vi "Buttons enable or disable.vi"(8 "error in (no error)":errorcluster, 10 "Enabled or Disabled?":T1(ring), 11 "Input references array":refnum<vi>[](array[refnum])) -> (0 "error out":errorcluster)   [LabVIEW 2014]
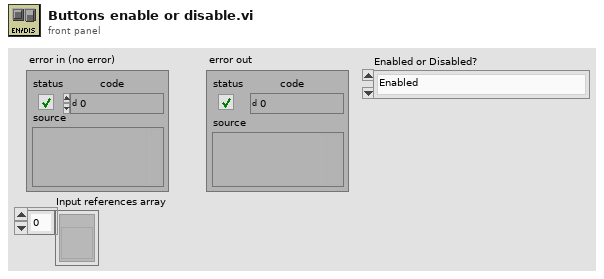
[diagram p1: front panel]
types:
  T1 = enum8{"Enabled", "Disabled", "Disabled and Grayed Out"}
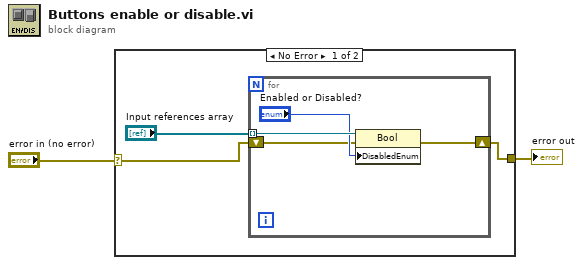
[diagram p0: block diagram]
diagram:
  n1 = case shown="No Error" "error in (no error)" {
    selector: "error in (no error)" -> [w4 w10]
    tunnel: [w3 w10] -> w1
    frame No Error {
      n2 = for {
        tunnel: "Input references array" -> [w9] mode=indexing
        shift-right: [w6] -> w3
        shift-left: w4 -> [w7]
        n3 = property class="Bool"(reference=w9, error in=w7, "DisabledEnum"="Enabled or Disabled?") -> (error out=w6:errorcluster)  [unwired: 1 out]
      }
    }
    frame Error {
    }
  }
  "error out" <- w1
